vi "LWXPS_ZygoWriteWord.vi"(0 "XPS Reference IN":refnum<k24>, 5 "Axis number":string, 7 "Register value":string, 9 "Data":string, 11 "LabVIEW error IN":errorcluster) -> (4 "XPS Reference OUT":refnum<k24>, 6 "Returned error code":i32, 8 "Response":string, 10 "XPS Error String":string, 15 "LabVIEW error OUT":errorcluster)   [LabVIEW 2014]
uses:
  D:/XPSQ8_LabView_Library/Development/Source/Dll/Newport.XPS.CommandInterface.dll
  Dll/Newport.XPS.CommandInterface.dll
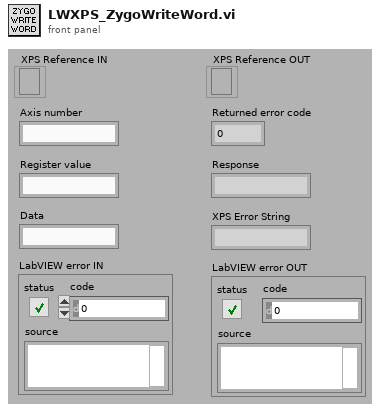
[diagram p1: front panel]
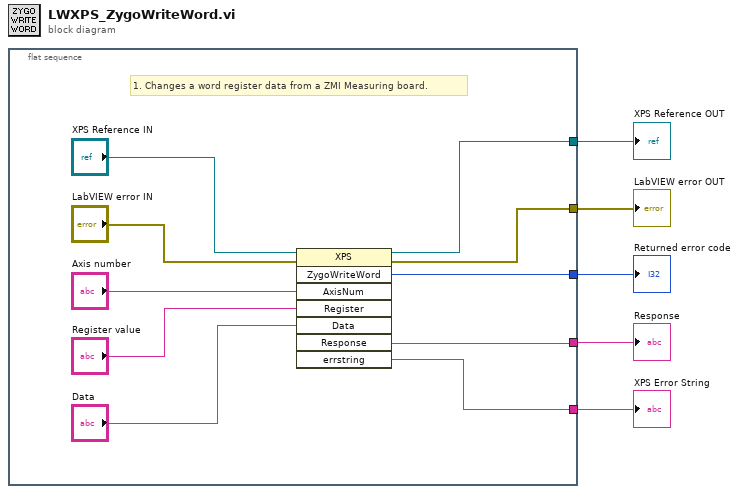
[diagram p0: block diagram]
diagram:
  n1 = flat-sequence {
    tunnel: [w13] -> w5
    tunnel: [w10] -> w4
    tunnel: [w14] -> w3
    tunnel: [w7] -> w2
    tunnel: [w8] -> w1
    frame #0 {
      # "1. Changes a word register data from a ZMI Measuring board."
      n2 = invoke class="XPS" method="ZygoWriteWord"(reference="XPS Reference IN", error in="LabVIEW error IN", "AxisNum"="Axis number", "Register"="Register value", "Data"="Data") -> (reference out=w13:refnum<k24>, error out=w10:errorcluster, "ZygoWriteWord"=w14:i32, "Response"=w8:string, "errstring"=w7:string)  [unwired: 3 in, 3 out]
    }
  }
  "XPS Reference OUT" <- w5
  "LabVIEW error OUT" <- w4
  "Returned error code" <- w3
  "XPS Error String" <- w2
  "Response" <- w1
